vi "Renishaw-XL80_SetUpdateAirCompMethod2.vi"(6 "Pressure [Pa]":dbl, 8 "error in (no error)":errorcluster, 9 "Humidity [%]":dbl, 10 "Air Temp [°C]":dbl, 11 "Renishaw-XL80 in":refnum<class "Renishaw-XL80.lvclass">) -> (0 "error out":errorcluster, 3 "Renishaw-XL80 out":refnum<class "Renishaw-XL80.lvclass">)   [LabVIEW 2024, in "Renishaw-XL80.lvclass"]
doc: "This method updates lambda using supplied values for air temperature (oC), air pressure (Pa), and air humidity (%RH).\n\nDefinition\nHRESULTUpdateAirComp2(\n [in] double dAirTemp,\n [in] double dPressure,\n [in] double dHumidity\n);\nParameters\ndAirTemp\nA variable that specifies the air temperature (in oC).\n\ndPressure\nA variable that specifies the air pressure (in Pa).\n\ndHumidity\nA variable that specifies the air humidity (in %RH).\n\nComments\nThis method will return with an HRESULT of E_FAIL if AutoCompensationMode is not set to AUTO_COMPENSATION_OFF. This warns the client that calculating Lambda whilst it is being automatically updated is somewhat pointless.\n\nIf successful this method will return an HRESULT of S_OK."
uses:
  Renishaw-XL80.lvclass
  Renishaw-XL80.lvclass/Renishaw-XL80.ctl
  D:/A.C.M/Example CSharp_64/bin/Debug/Interop.DX10SDKADAPTORLib.dll
  Example CSharp_64/bin/Debug/Interop.DX10SDKADAPTORLib.dll
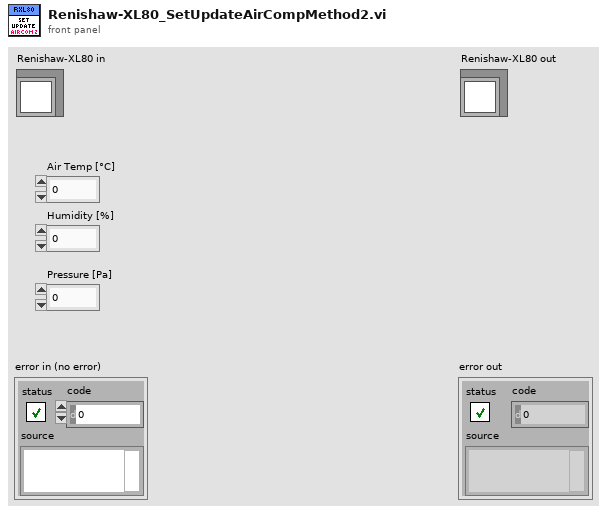
[diagram p1: front panel]
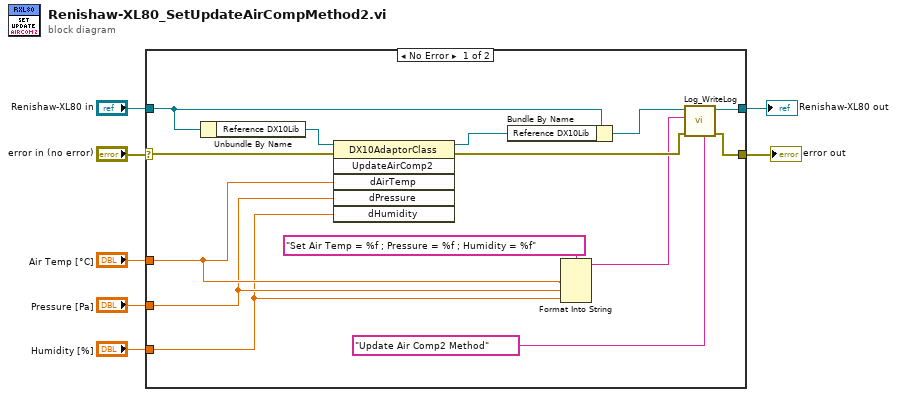
[diagram p0: block diagram]
diagram:
  n1 = case shown="No Error" "error in (no error)" {
    selector: "error in (no error)" -> [w14 w23]
    tunnel: [w13 w23] -> w6
    tunnel: [w15 w22] -> w4
    tunnel: "Renishaw-XL80 in" -> [w16 w22]
    tunnel: "Humidity [%]" -> [w9 _]
    tunnel: "Air Temp [°C]" -> [w11 _]
    tunnel: "Pressure [Pa]" -> [w10 _]
    frame No Error {
      n2 = Unbundle By Name(w16) -> ("Reference DX10Lib"=w21:refnum<k24>)
      n3 = invoke class="DX10AdaptorClass" method="UpdateAirComp2"(reference=w21, error in=w14, "dAirTemp"=w11, "dPressure"=w10, "dHumidity"=w9) -> (reference out=w19:refnum<k24>, error out=w18:errorcluster)  [unwired: 1 in, 4 out]
      n4 = Bundle By Name(cluster=w16, "Reference DX10Lib"=w19) -> (w20:refnum<class "Renishaw-XL80.lvclass">)
      n5 = Format Into String(format string="Set Air Temp = %f ; Pressure = %f ; Humidity = %f", w11, w10, w9) -> (resulting string=w8:string)  [unwired: 2 in, 1 out]
      n6 = call-dynamic "Log_WriteLog.vi"("Additional text"="Update Air Comp2 Method", "error in (no error)"=w18, "Command"=w8, "Log in"=w20) -> ("error out"=w13:errorcluster, "Log out"=w15:refnum<class "Renishaw-XL80.lvclass">)  [unwired: 6 in]
    }
    frame Error {
    }
  }
  "error out" <- w6
  "Renishaw-XL80 out" <- w4
